vi "InitMatlabEnv.vi"(8 "Matlab Working Directory":path, 10 "matlab src":path, 11 "MatlabSystemPath":path) -> ()   [LabVIEW 2017]
uses:
  Globals/gloablDefinitions.vi
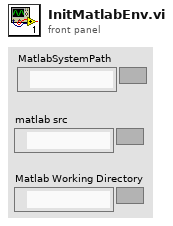
[diagram p1: front panel]
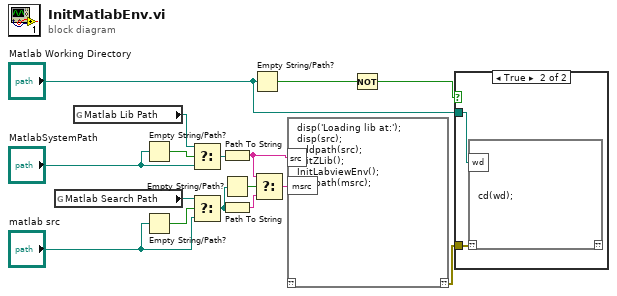
[diagram p0: block diagram]
diagram:
  n1 = global read "gloablDefinitions.vi" "Matlab Search Path"() -> (w7:path)
  n2 = global read "gloablDefinitions.vi" "Matlab Lib Path"() -> (w11:path)
  n3 = Empty String/Path?(string/path="MatlabSystemPath") -> (empty?=w12:bool)
  n4 = Empty String/Path?(string/path="matlab src") -> (empty?=w8:bool)
  n5 = Select(t=w11, s=w12, f="MatlabSystemPath") -> (s? t:f=w9:path)
  n6 = Select(t=w7, s=w8, f="matlab src") -> (s? t:f=w5:path)
  n7 = Path To String(path=w9) -> (string=w14:string)
  n8 = Empty String/Path?(string/path=w5) -> (empty?=w16:bool)
  n9 = Path To String(path=w5) -> (string=w15:string)
  n10 = Empty String/Path?(string/path="Matlab Working Directory") -> (empty?=w4:bool)
  n11 = Select(t=w14, s=w16, f=w15) -> (s? t:f=w13:string)
  n12 = script code="disp('Loading lib at:');\ndisp(src);\naddpath(src);\nInitZLib();\nInitLabviewEnv();\naddpath(msrc);"("src"=w14, "msrc"=w13) -> ("??"=w1:errorcluster)  [unwired: 1 in]
  n13 = Not(x=w4) -> (.not. x?=w3:bool)
  n14 = case shown="True" w3 {
    tunnel: "Matlab Working Directory" -> [_ w18]
    tunnel: w1 -> [_ w17]
    frame False {
    }
    frame True {
      n15 = script code="cd(wd);"("??"=w17, "wd"=w18) -> ()  [unwired: 1 out]
    }
  }
